vi "controller demo.vi"() -> ()   [LabVIEW 2013]
uses:
  <vilib>/Utility/inputDevices.llb/closeJoystick.vi
  <vilib>/Utility/inputDevices.llb/joystickAcquire.vi
panel:
  out "Start":bool
  out "Back":bool
  out "Right Front Top":bool
  out "Left Front Top":bool
  out "Button Y":bool
  out "Button X":bool
  out "Button B":bool
  out "Pivot degrees":i32
  out "Right stick\nTop / Bottom":i32
  out "Right stick\nLeft / Right":i32
  out "Button A":bool
  out "Front\nLeft / Right":i32
  out "Left stick\nTop / Bottom":i32
  out "Left stick\nLeft / Right":i32
  in  "stop":bool
  out "error out":errorcluster
  # "This VI demonstrates the use of a Logitech F310 controller.  Mode button should be OFF and Interface button should be on X."
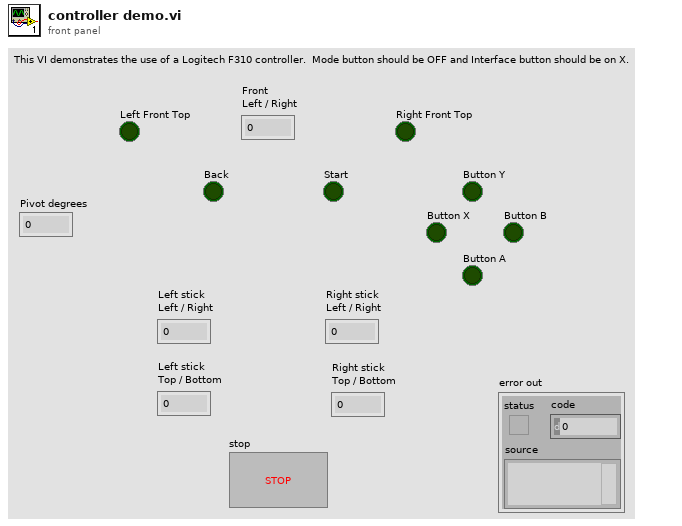
[diagram p1: front panel]
types:
  T1 = cluster{"X axis":i32, "Y axis":i32, "Z axis":i32, "X axis rotation":i32, "Y axis rotation":i32, "Z axis rotation":i32, "U axis":i32, "V axis":i32}
  T2 = cluster{"button 1":bool, "button 2":bool, "button 3":bool, "button 4":bool, "button 5":bool, "button 6":bool, "button 7":bool, "button 8":bool, "button 9":bool, "button 10":bool, "button 11":bool, "button 12":bool, "button 13":bool, "button 14":bool, "button 15":bool, "button 16":bool, "button 17":bool, "button 18":bool, "button 19":bool, "button 20":bool, "button 21":bool, "button 22":bool, "button 23":bool, "button 24":bool, "button 25":bool, "button 26":bool, "button 27":bool, "button 28":bool, "button 29":bool, "button 30":bool, "button 31":bool, "button 32":bool}
  T3 = cluster{"pov 1":i32, "pov 2":i32, "pov 3":i32, "pov 4":i32}
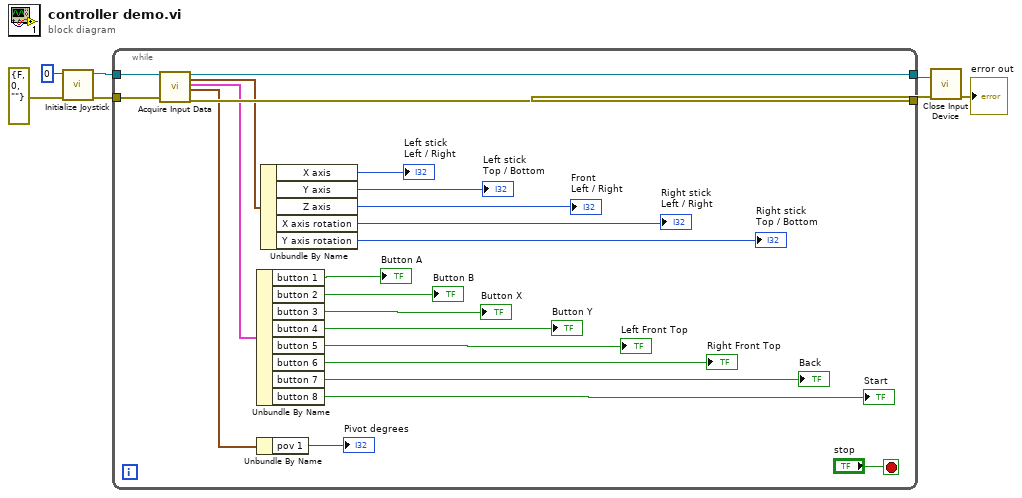
[diagram p0: block diagram]
diagram:
  n1 = call <vilib>:"Initialize Joystick.vi"("error in (no error)"=errorcluster {"status"=FALSE, "code"=0, "source"=""}, "device index"=0) -> ("error out"=w3:errorcluster, "device ID"=w6:refnum<k1>)  [unwired: 8 in]
  n2 = while {
    tunnel: w6 -> [w29]
    tunnel: [w28] -> w5
    tunnel: w3 -> [w27]
    tunnel: [w26] -> w2
    stop <- "stop" stop-if-true
    n3 = call-poly <vilib>:"Acquire Input Data.vi"("device ID"=w29, "error in (no error)"=w27) -> ("device ID"=w28:refnum<k1>, "axis info"=w25:T1, "button info"=w23:T2, "direction info"=w22:T3, "error out"=w26:errorcluster)  [unwired: 13 in]
    n4 = Unbundle By Name(w23) -> ("button 1"=→"Button A":bool, "button 2"=→"Button B":bool, "button 3"=→"Button X":bool, "button 4"=→"Button Y":bool, "button 5"=→"Left Front Top":bool, "button 6"=→"Right Front Top":bool, "button 7"=→"Back":bool, "button 8"=→"Start":bool)
    n5 = Unbundle By Name(w22) -> ("pov 1"=→"Pivot degrees":i32)
    n6 = Unbundle By Name(w25) -> ("X axis"=→"Left stick\nLeft / Right":i32, "Y axis"=→"Left stick\nTop / Bottom":i32, "Z axis"=→"Front\nLeft / Right":i32, "X axis rotation"=→"Right stick\nLeft / Right":i32, "Y axis rotation"=→"Right stick\nTop / Bottom":i32)
  }
  n7 = call-poly <vilib>:"Close Input Device.vi"("error in (no error)"=w2, "device ID"=w5) -> ("error out"=→"error out":errorcluster)  [unwired: 8 in]
